vi "BesselJ_CDB.vi"(1 "n":i32, 2 "a+bi":cdb=1.0+1.0i) -> (0 "Jn(a+bi)":cdb=0.9376084768060292-0.49652994760912217i format="%#.14g")   [LabVIEW 2011]
uses:
  <vilib>/Analysis/2dsp.llb/Integral Method.ctl
  <vilib>/Analysis/8numeric.llb/1D Numeric Integration.vi
  <vilib>/Analysis/1siggen.llb/Ramp Pattern by Delta.vi
  <vilib>/Analysis/NI_AALBase.lvlib
  <vilib>/Analysis/NI_AALPro.lvlib
panel:
  in  "n Intervals":i32=20
  # "Paul Nathan 18/10/2011"
  # "Tests revealed that >20 steps DECREASES accuracy!"
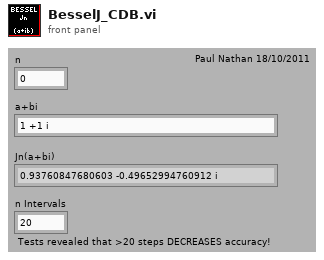
[diagram p1: front panel]
types:
  T1 = typedef "NI_AALPro.lvlib/Integral Method.ctl" = i32
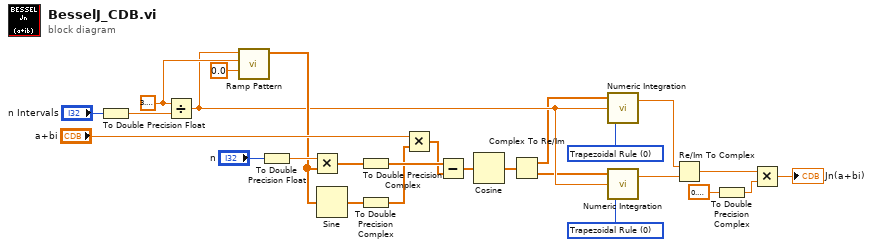
[diagram p0: block diagram]
diagram:
  w10 = T1 0 items=["Trapezoidal Rule", "Simpson's Rule", "Simpson's 3/8 Rule", "Bode Rule"] ("integration method")
  w11 = T1 0 items=["Trapezoidal Rule", "Simpson's Rule", "Simpson's 3/8 Rule", "Bode Rule"] ("integration method")
  w25 = 3.141592653589793
  n1 = To Double Precision Float(number="n Intervals") -> (double precision float=w23:dbl)
  n2 = Divide(x=w25, y=w23) -> (x/y=w9:dbl)
  n3 = call-poly <vilib>:"Ramp Pattern.vi"("start"=0.0, "end"=w25, "delta"=w9) -> ("Ramp Pattern"=w14:dbl[])  [unwired: 6 in, 2 out]
  n4 = To Double Precision Float(number="n") -> (double precision float=w15:dbl)
  n5 = Multiply(x=w15, y=w14) -> (x*y=w21:dbl[])
  n6 = Sine(x=w14) -> (sin(x)=w19:dbl[])
  n7 = To Double Precision Complex(1:w21) -> (0:w20:cdb[])
  n8 = To Double Precision Complex(1:w19) -> (0:w17:cdb[])
  n9 = Multiply(x="a+bi", y=w17) -> (x*y=w16:cdb[])
  n10 = Subtract(x=w20, y=w16) -> (x-y=w13:cdb[])
  n11 = Cosine(x=w13) -> (cos(x)=w12:cdb[])
  n12 = Complex To Re/Im(x + iy=w12) -> (x=w2:dbl[], y=w1:dbl[])
  n13 = call-poly <vilib>:"Numeric Integration.vi"("integration method"=w11, "dt"=w9, "Input Array"=w2) -> ("result"=w8:dbl)  [unwired: 1 out]
  n14 = call-poly <vilib>:"Numeric Integration.vi"("integration method"=w10, "dt"=w9, "Input Array"=w1) -> ("result"=w7:dbl)  [unwired: 1 out]
  n15 = Re/Im To Complex(1:w7, 2:w8) -> (0:w6:cdb)
  n16 = To Double Precision Complex(1:0.3183098861837907) -> (0:w4:cdb)
  n17 = Multiply(x=w6, y=w4) -> (x*y=→"Jn(a+bi)":cdb)
